vi "PhotonPoseEstimator_GetEmptyPose.vi"() -> (3 "EmptyPose":T1={"Translation3d"={"X"=0.0, "Y"=0.0, "Z"=0.0}, "Rotation3d"={"Q_quaternion"={"R"=1.0, "V"=[0.0, 0.0, 0.0]}}} {"Translation3d"."Z" format="%14.3f"; "Translation3d"."Y" format="%14.3f"; "Translation3d"."X" format="%14.3f"})   [LabVIEW 2019, in "PhotonVisionLib.lvlib"]
uses:
  <vilib>/Rock Robotics/WPI/ThirdParty/JAS_Junk/TrajLib/TypeDef/POSE3D.ctl
  <vilib>/Rock Robotics/WPI/ThirdParty/JAS_Junk/TrajLib/TypeDef/TRANSLATION3D.ctl
  <vilib>/Rock Robotics/WPI/ThirdParty/JAS_Junk/TrajLib/TypeDef/ROTATION3D.ctl
  <vilib>/Rock Robotics/WPI/ThirdParty/JAS_Junk/TrajLib/TypeDef/QUATERNION.ctl
  PhotonVisionLib.lvlib
  <vilib>/Rock Robotics/WPI/ThirdParty/JAS_Junk/TrajLib/Trajectory_Library.lvlib
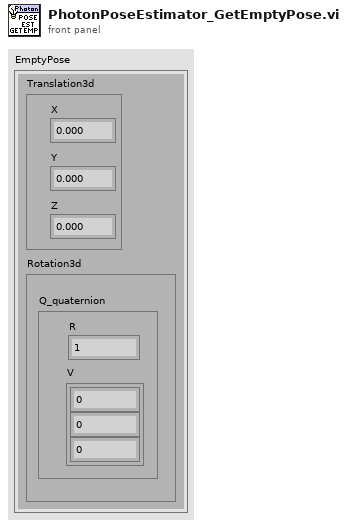
[diagram p1: front panel]
types:
  T1 = typedef "Trajectory_Library.lvlib/POSE3D.ctl" = cluster{"Translation3d":T2, "Rotation3d":T3}
  T2 = typedef "Trajectory_Library.lvlib/TRANSLATION3D.ctl" = cluster{"X":dbl, "Y":dbl, "Z":dbl}
  T3 = typedef "Trajectory_Library.lvlib/ROTATION3D.ctl" = cluster{"Q_quaternion":T4}
  T4 = typedef "Trajectory_Library.lvlib/QUATERNION.ctl" = cluster{"R":dbl, "V":dbl[]}
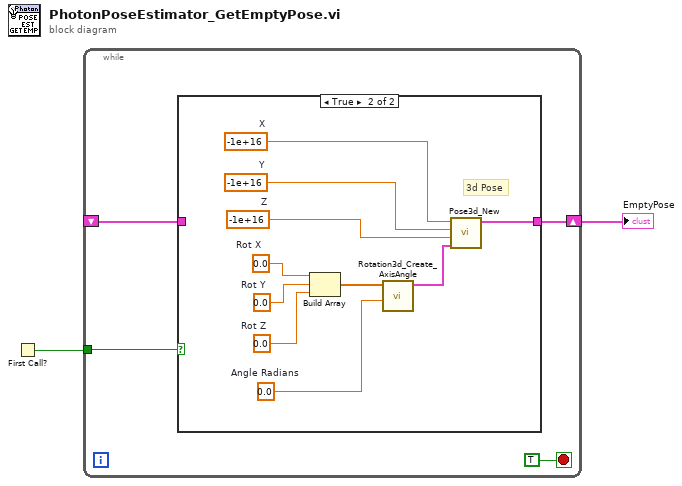
[diagram p0: block diagram]
diagram:
  n1 = First Call?() -> (First Call?: T/F=w2:bool)
  n2 = while {
    tunnel: w2 -> [w5]
    shift-right: [w4] -> w1
    shift-left: _ -> [w3]
    stop <- TRUE stop-if-true
    n3 = case shown="True" w5 {
      tunnel: [w7 w8] -> w4
      tunnel: w3 -> [w7 _]
      frame False {
      }
      frame True {
        w16 = -1e+16  # X
        w15 = -1e+16  # Y
        w14 = -1e+16  # Z
        w12 = 0.0  # Rot Z
        w10 = 0.0  # Rot X
        w11 = 0.0  # Rot Y
        w17 = 0.0  # Angle Radians
        # "3d Pose"
        n4 = Build Array(w10, w11, w12) -> (w9:dbl[])
        n5 = call <vilib>:"Rotation3d_Create_AxisAngle.vi"("Angle"=w17, "Axis Vector"=w9) -> ("Rotation3d"=w13:T3)  [unwired: 9 in]
        n6 = call <vilib>:"Pose3d_New.vi"("Rotation3d"=w13, "z"=w14, "Y"=w15, "X"=w16) -> ("out Pose3d"=w8:T1)  [unwired: 7 in]
      }
    }
  }
  "EmptyPose" <- w1
